vi "SaveNewPAQtags.vi"(8 "error in (no error)":errorcluster, 10 "TAGpropertyEdit":T1 {"TAGprop"."TagFunc" format="%08x"; "TAGprop"."RangeL" format="%.2f"; "TAGprop"."RangeH" format="%.2f"}, 11 "DBAL-SQLite in":refnum<class "DBAL-SQLite.lvclass">) -> (0 "error out":errorcluster, 3 "DBAL-SQLite out":refnum<class "DBAL-SQLite.lvclass">)   [LabVIEW 2020, in "Sgraph_lib_V1.lvlib" / "DBAL-SQLite.lvclass"]
doc: "must Override!"
uses:
  DBAL-SQLite.lvclass
  controls/DBAL_TAGpropEdit.ctl
  Common/controls/typedef_com_TagProp.ctl
  DBAL.lvclass
  Builds/Sgraph_lib_V1.lvlib
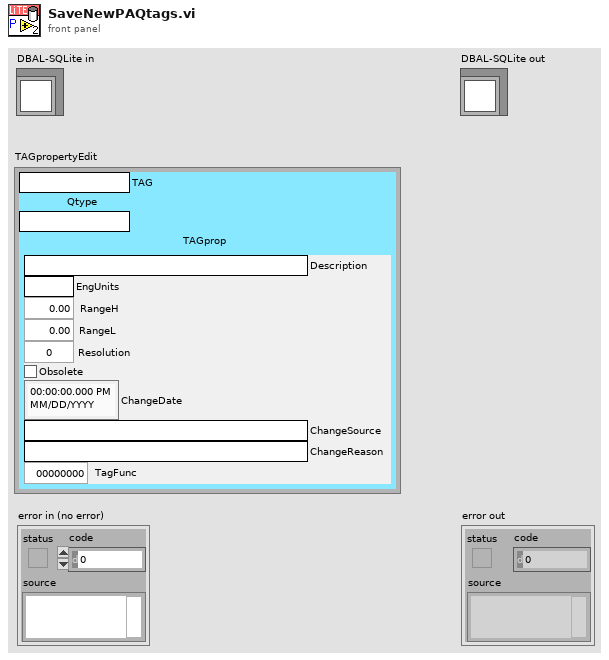
[diagram p1: front panel]
types:
  T1 = typedef "Sgraph_lib_V1.lvlib/DBAL.lvclass/DBAL_TAGpropEdit.ctl" = cluster{"TAG":string, "Qtype":string, "TAGprop":T2}
  T2 = typedef "Sgraph_lib_V1.lvlib/typedef_com_TagProp.ctl" = cluster{"Description":string, "EngUnits":string, "RangeH":dbl, "RangeL":dbl, "Resolution":i32, "Obsolete":bool, "ChangeDate":timestamp, "ChangeSource":string, "ChangeReason":string, "TagFunc":u32}
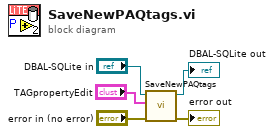
[diagram p0: block diagram]
diagram:
  n1 = call-parent "SaveNewPAQtags.vi"("error in (no error)"="error in (no error)", "TAGpropertyEdit"="TAGpropertyEdit", "DBAL in"="DBAL-SQLite in") -> ("error out"=→"error out":errorcluster, "DBAL out"=→"DBAL-SQLite out":refnum<class "DBAL-SQLite.lvclass">)  [unwired: 7 in]
